vi "SwerveAngleEncoderConversion.vi"(11 "Voltages":dbl[](array[numeric])) -> (3 "Angles":dbl[](array[numeric]))   [LabVIEW 2018]
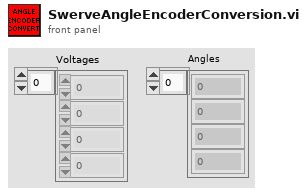
[diagram p1: front panel]
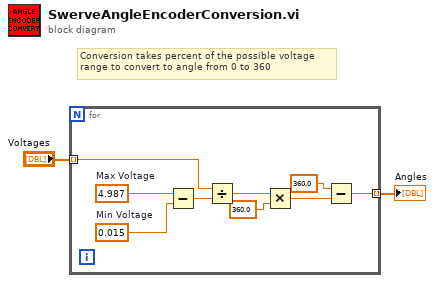
[diagram p0: block diagram]
diagram:
  # "Conversion takes percent of the possible voltage\nrange to convert to angle from 0 to 360"
  n1 = for {
    tunnel: "Voltages" -> [w3] mode=indexing
    tunnel: [w11] -> w1 mode=indexing
    w5 = 0.015  # Min Voltage
    w6 = 4.987  # Max Voltage
    n2 = Subtract(x=w6, y=w5) -> (x-y=w4:dbl)
    n3 = Divide(x=w3, y=w4) -> (x/y=w10:dbl)
    n4 = Multiply(x=w10, y=360.0) -> (x*y=w7:dbl)
    n5 = Subtract(x=360.0, y=w7) -> (x-y=w11:dbl)
  }
  "Angles" <- w1
